vi "GetLogContent.vi"(8 "error in (no error)":errorcluster, 11 "GenericCanAdapterClass in":refnum<class "GenericCanAdapterClass.lvclass">) -> (0 "error out":errorcluster, 2 "LogContent":string[](array[string]), 3 "GenericCanAdapterClass out":refnum<class "GenericCanAdapterClass.lvclass">)   [LabVIEW 2011, in "GenericCanAdapterClass.lvclass"]
uses:
  GenericCanAdapterClass.lvclass
  GenericCanAdapterClass.lvclass/GenericCanAdapterClass.ctl
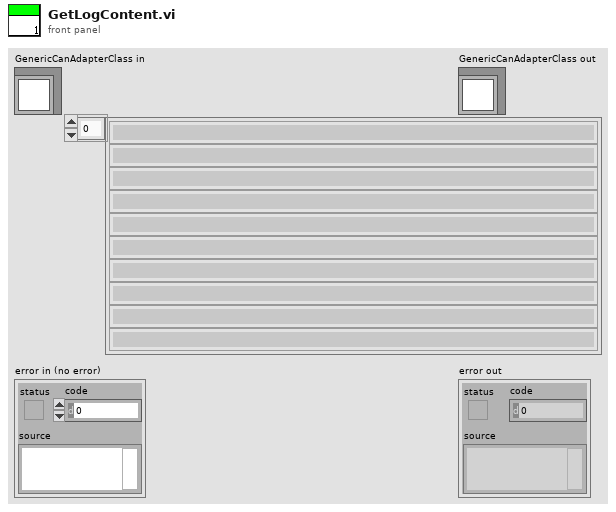
[diagram p1: front panel]
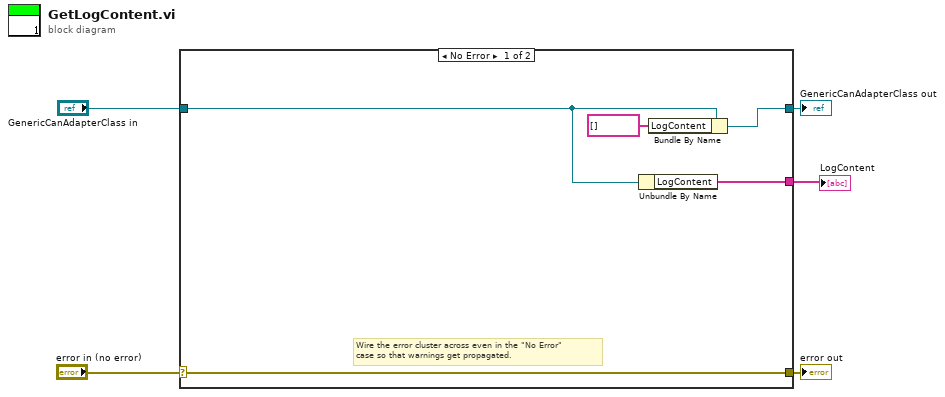
[diagram p0: block diagram]
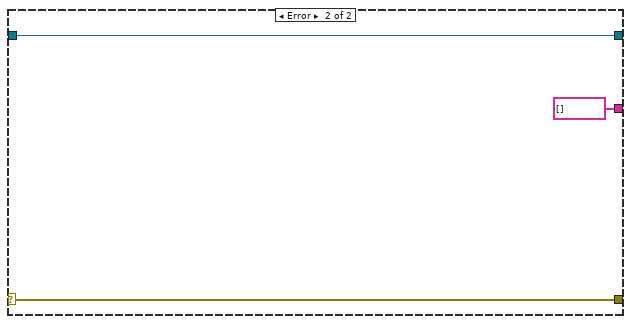
[diagram p2: hidden frame]
diagram:
  n1 = case shown="No Error" "error in (no error)" {
    selector: "error in (no error)" -> [w10 w13]
    tunnel: [w10 w13] -> w4
    tunnel: [w7 w12] -> w2
    tunnel: "GenericCanAdapterClass in" -> [w8 w12]
    tunnel: [w9 string[] [] ("LogContent")] -> w1
    frame No Error {
      # "Wire the error cluster across even in the \"No Error\"\ncase so that warnings get propagated."
      n2 = Unbundle By Name(w8) -> ("LogContent"=w9:string[])
      n3 = Bundle By Name(cluster=w8, "LogContent"=string[] []) -> (w7:refnum<class "GenericCanAdapterClass.lvclass">)
    }
    frame Error {
    }
  }
  "error out" <- w4
  "GenericCanAdapterClass out" <- w2
  "LogContent" <- w1
